vi "GetLoadedInst.vi"(8 "error in (no error)":errorcluster caption="entrée d'erreur (pas d'erreur)", 11 "Experiment en entrée":refnum<class "Experiment.lvclass">) -> (0 "error out":errorcluster caption="sortie d'erreur", 2 "LoadedInst":refnum<class "BaseDevice.lvclass">[](array[class]), 3 "Experiment en sortie":refnum<class "Experiment.lvclass">)   [LabVIEW 2019, in "Experiment.lvclass"]
uses:
  Experiment.lvclass
  DevicesClass/BaseDevice/BaseDevice.lvclass
  Experiment.lvclass/Experiment.ctl
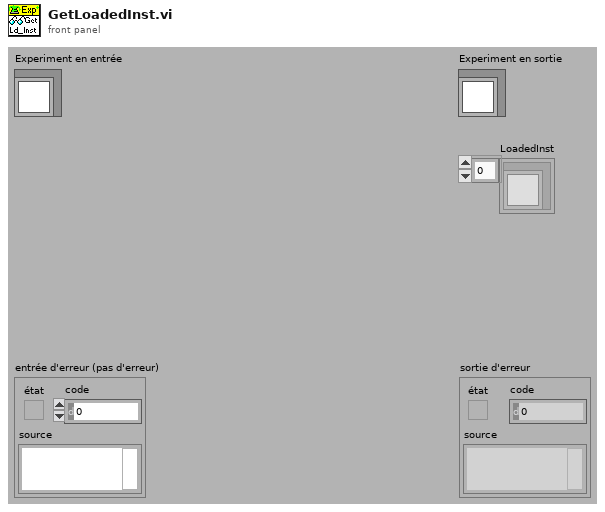
[diagram p1: front panel]
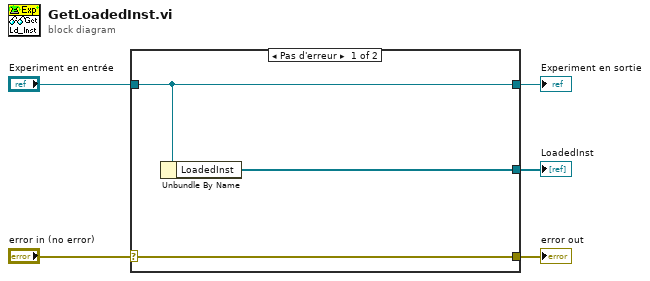
[diagram p0: block diagram]
diagram:
  n1 = case shown="Pas d'erreur" "error in (no error)" {
    selector: "error in (no error)" -> [w8 w9]
    tunnel: [w8 w9] -> w4
    tunnel: [w7 w10] -> w2
    tunnel: "Experiment en entrée" -> [w7 w10]
    tunnel: [w6 _] -> w1
    frame No Error {
      n2 = Unbundle By Name(w7) -> ("LoadedInst"=w6:refnum<class "BaseDevice.lvclass">[])
    }
    frame Error {
    }
  }
  "error out" <- w4
  "Experiment en sortie" <- w2
  "LoadedInst" <- w1
